vi "ChangePaneOriginToPosition.vi"(8 "error in (no error)":errorcluster, 9 "New Origin":T1, 10 "Pane":u16(ring) items=["Top", "Left", "Center", "Right", "Bottom"], 11 "PentaPanesGUI in":refnum<class "PentaPanes.lvclass">) -> (0 "error out":errorcluster, 3 "PentaPanesGUI out":refnum<class "PentaPanes.lvclass">)   [LabVIEW 2022 SP3, in "PentaPanesLibrary.lvlib" / "PentaPanes.lvclass"]
doc: "This VI reads the Pane's position string and Label.\n\nPaneRef - A reference to the pane. \nPos String - Outputs a position string (\"Top\", \"Left\", \"Right\", \"Bottom\").\nLabel.Text - Outputs The Label of the pane."
uses:
  PentaPanes.lvclass
  <vilib>/Utility/miscctls.llb/LVPointTypeDef.ctl
  PentaPanes.lvclass/PentaPanes.ctl
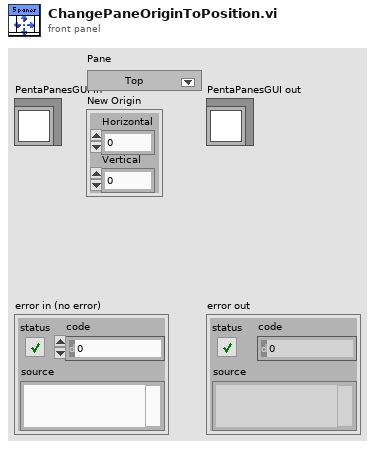
[diagram p1: front panel]
types:
  T1 = typedef "LVPointTypeDef.ctl" = cluster{"Horizontal":i16, "Vertical":i16}
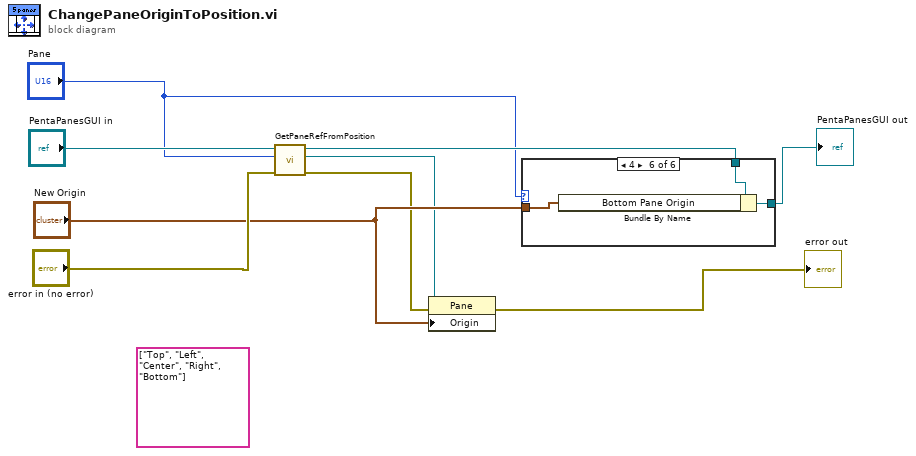
[diagram p0: block diagram]
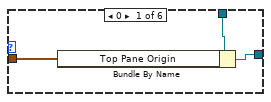
[diagram p2: hidden frame]
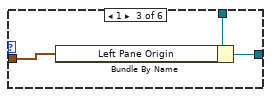
[diagram p4: hidden frame]
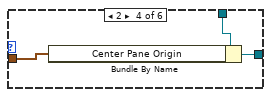
[diagram p5: hidden frame]
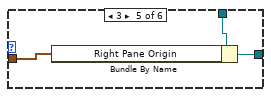
[diagram p6: hidden frame]
diagram:
  (unwired) string[] ["Top", "Left", "Center", "Right", "Bottom"]
  n1 = call "GetPaneRefFromPosition.vi"("error in (no error)"="error in (no error)", "Position"="Pane", "PentaPanesGUI in"="PentaPanesGUI in") -> ("error out"=w2:errorcluster, "PaneRef"=w3:refnum<vi>, "PentaPanesGUI out"=w7:refnum<class "PentaPanes.lvclass">)  [unwired: 6 in]
  n2 = property class="Pane"(reference=w3, error in=w2, "Origin"="New Origin") -> (error out=→"error out":errorcluster)  [unwired: 1 out]
  n3 = case shown="4" "Pane" {
    tunnel: w7 -> [w12 w13 w16 w19 w22 w25]
    tunnel: "New Origin" -> [w11 _ w15 w18 w21 w24]
    tunnel: [w10 w13 w14 w17 w20 w23] -> w6
    frame 0 {
      n4 = Bundle By Name(cluster=w12, "Top Pane Origin"=w11) -> (w10:refnum<class "PentaPanes.lvclass">)
    }
    frame 5, Default {
    }
    frame 1 {
      n5 = Bundle By Name(cluster=w16, "Left Pane Origin"=w15) -> (w14:refnum<class "PentaPanes.lvclass">)
    }
    frame 2 {
      n6 = Bundle By Name(cluster=w19, "Center Pane Origin"=w18) -> (w17:refnum<class "PentaPanes.lvclass">)
    }
    frame 3 {
      n7 = Bundle By Name(cluster=w22, "Right Pane Origin"=w21) -> (w20:refnum<class "PentaPanes.lvclass">)
    }
    frame 4 {
      n8 = Bundle By Name(cluster=w25, "Bottom Pane Origin"=w24) -> (w23:refnum<class "PentaPanes.lvclass">)
    }
  }
  "PentaPanesGUI out" <- w6
